vi "PGSetChannelMode.vi"(8 "error in":errorcluster, 11 "VISA resource name":refnum<visa-resource-name>="COM7") -> (0 "error out":errorcluster, 3 "VISA resource name out":refnum<visa-resource-name>)   [LabVIEW 2018]
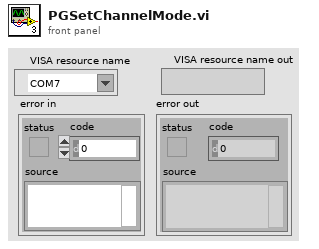
[diagram p1: front panel]
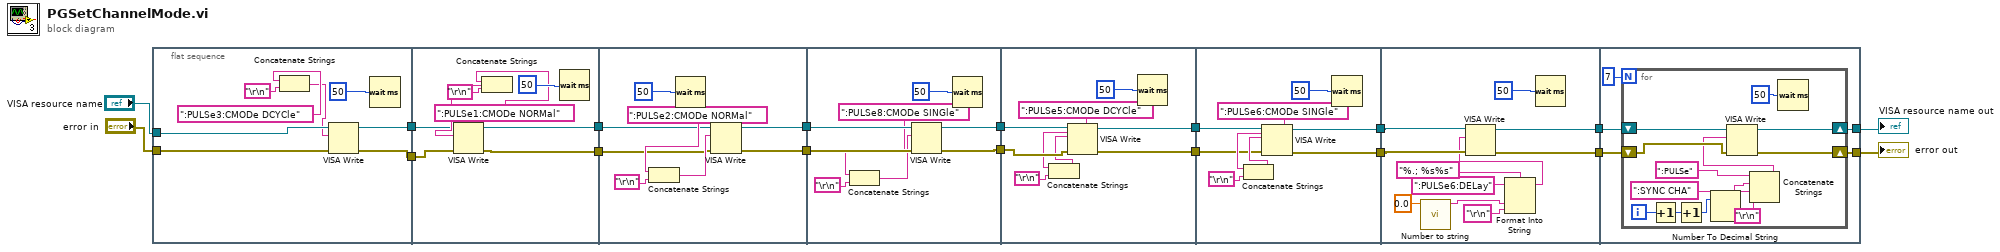
[diagram p0: block diagram]
diagram:
  n1 = flat-sequence {
    tunnel: "error in" -> [w25]
    tunnel: "VISA resource name" -> [w24]
    tunnel: [w20] -> w8
    tunnel: [w19] -> w7
    tunnel: [w30] -> w10
    tunnel: [w29] -> w9
    tunnel: w8 -> [w28]
    tunnel: w7 -> [w27]
    tunnel: [w42] -> w18
    tunnel: [w41] -> w17
    tunnel: w10 -> [w36]
    tunnel: w9 -> [w35]
    tunnel: w18 -> [w50]
    tunnel: w17 -> [w49]
    tunnel: [w47] -> w14
    tunnel: [w46] -> w13
    tunnel: w14 -> [w58]
    tunnel: w13 -> [w57]
    tunnel: [w56] -> w12
    tunnel: [w55] -> w11
    tunnel: w12 -> [w61]
    tunnel: w11 -> [w62]
    tunnel: [w60] -> w5
    tunnel: [w59] -> w4
    tunnel: w5 -> [w75]
    tunnel: w4 -> [w76]
    tunnel: [w74] -> w2
    tunnel: [w73] -> w1
    tunnel: [w78] -> w3
    tunnel: [w79] -> w6
    tunnel: w2 -> [w80]
    tunnel: w1 -> [w81]
    frame #0 {
      n2 = Concatenate Strings(":PULSe3:CMODe DCYCle" ("write buffer"), "\r\n") -> (w21:string)
      n3 = VISA Write(VISA resource name=w24, write buffer=w21, error in (no error)=w25) -> (VISA resource name out=w19:refnum<visa-resource-name>, error out=w20:errorcluster)  [unwired: 1 out]
      n4 = Wait (ms)(milliseconds to wait=50) -> ()  [unwired: 1 out]
    }
    frame #1 {
      n5 = Concatenate Strings(":PULSe1:CMODe NORMal" ("write buffer"), "\r\n") -> (w31:string)
      n6 = VISA Write(VISA resource name=w27, write buffer=w31, error in (no error)=w28) -> (VISA resource name out=w30:refnum<visa-resource-name>, error out=w29:errorcluster)  [unwired: 1 out]
      n7 = Wait (ms)(milliseconds to wait=50) -> ()  [unwired: 1 out]
    }
    frame #2 {
      n8 = Concatenate Strings(":PULSe2:CMODe NORMal" ("write buffer"), "\r\n") -> (w37:string)
      n9 = Wait (ms)(milliseconds to wait=50) -> ()  [unwired: 1 out]
      n10 = VISA Write(VISA resource name=w36, write buffer=w37, error in (no error)=w35) -> (VISA resource name out=w41:refnum<visa-resource-name>, error out=w42:errorcluster)  [unwired: 1 out]
    }
    frame #3 {
      n11 = Concatenate Strings(":PULSe8:CMODe SINGle" ("write buffer"), "\r\n") -> (w43:string)
      n12 = VISA Write(VISA resource name=w49, write buffer=w43, error in (no error)=w50) -> (VISA resource name out=w47:refnum<visa-resource-name>, error out=w46:errorcluster)  [unwired: 1 out]
      n13 = Wait (ms)(milliseconds to wait=50) -> ()  [unwired: 1 out]
    }
    frame #4 {
      n14 = Concatenate Strings(":PULSe5:CMODe DCYCle" ("write buffer"), "\r\n") -> (w51:string)
      n15 = VISA Write(VISA resource name=w58, write buffer=w51, error in (no error)=w57) -> (VISA resource name out=w55:refnum<visa-resource-name>, error out=w56:errorcluster)  [unwired: 1 out]
      n16 = Wait (ms)(milliseconds to wait=50) -> ()  [unwired: 1 out]
    }
    frame #5 {
      n17 = Concatenate Strings(":PULSe6:CMODe SINGle" ("write buffer"), "\r\n") -> (w63:string)
      n18 = VISA Write(VISA resource name=w62, write buffer=w63, error in (no error)=w61) -> (VISA resource name out=w60:refnum<visa-resource-name>, error out=w59:errorcluster)  [unwired: 1 out]
      n19 = Wait (ms)(milliseconds to wait=50) -> ()  [unwired: 1 out]
    }
    frame #6 {
      n20 = call "Number to string.vi"("Numeric"=0.0) -> ("Shortest String"=w67:string)  [unwired: 10 in]
      n21 = Format Into String(format string="%.; %s%s", initial string=":PULSe6:DELay" ("format string"), w67, "\r\n" ("format string")) -> (resulting string=w70:string)  [unwired: 1 in, 1 out]
      n22 = VISA Write(VISA resource name=w75, write buffer=w70, error in (no error)=w76) -> (VISA resource name out=w74:refnum<visa-resource-name>, error out=w73:errorcluster)  [unwired: 1 out]
      n23 = Wait (ms)(milliseconds to wait=50) -> ()  [unwired: 1 out]
    }
    frame #7 {
      n24 = for {
        N: 7 -> [_]
        shift-right: [w89] -> w79
        shift-left: w80 -> [w92]
        shift-right: [w90] -> w78
        shift-left: w81 -> [w91]
        i -> [w95]
        n25 = Increment(x=w95) -> (x+1=w94:i32)
        n26 = Increment(x=w94) -> (x+1=w93:i32)
        n27 = Number To Decimal String(number=w93) -> (decimal integer string=w87:string)  [unwired: 1 in]
        n28 = Concatenate Strings(":PULSe" ("string"), w87, ":SYNC CHA" ("string"), "\r\n") -> (w83:string)
        n29 = VISA Write(VISA resource name=w92, write buffer=w83, error in (no error)=w91) -> (VISA resource name out=w89:refnum<visa-resource-name>, error out=w90:errorcluster)  [unwired: 1 out]
        n30 = Wait (ms)(milliseconds to wait=50) -> ()  [unwired: 1 out]
      }
    }
  }
  "error out" <- w3
  "VISA resource name out" <- w6
